vi "Configure Channel.vi"(0 "VISA resource name":refnum<visa-resource-name>, 1 "Enable Channel (T: Enable)":bool=TRUE, 2 "Input Impedance (0: 1M ohm)":u16(ring) items=["1M", "50"], 3 "Bandwidth (0: FULL)":u16(ring) items=["FULL", "500 MHz", "250 MHz", "150 MHz", "20 MHz"], 5 "Channel (0: Channel 1)":u16(ring) format="%#_5f" items=["Channel 1", "Channel 2", "Channel 3", "Channel 4", "Math 1", "Math 2", "Math 3", "Math 4", "Reference 1", "Reference 2", "Reference 3", "Reference 4"], 7 "Vertical Coupling (1: DC)":u16(ring)=1 items=["AC", "DC", "Ground"], 9 "Probe Attenuation (1.0)":dbl=1.0, 11 "error in (no error)":errorcluster, 12 "Vertical Range (10.0 V)":dbl=10.0, 13 "Vertical Offset (0.0 V)":dbl) -> (4 "VISA resource name out":refnum<visa-resource-name>, 15 "error out":errorcluster)   [LabVIEW 2015, in "Tektronix 7000 Series.lvlib"]
doc: "Configures the vertical properties of an oscilloscope for a specified channel. \n\n<B>Note:</B> \nThis VI does not configure channel settings for disabled channels."
uses:
  Tektronix 7000 Series.lvlib
panel:
  # "Input Channel Parameters"
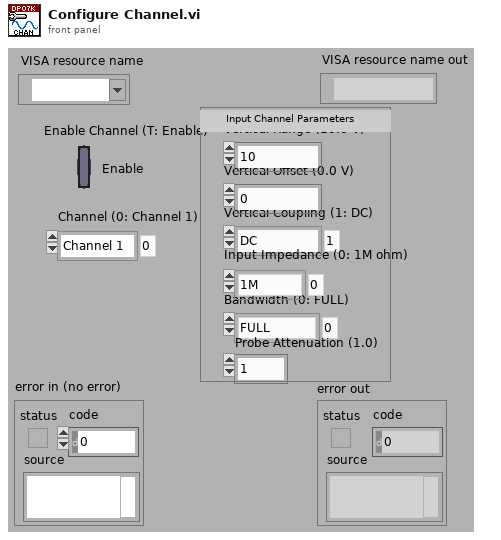
[diagram p1: front panel]
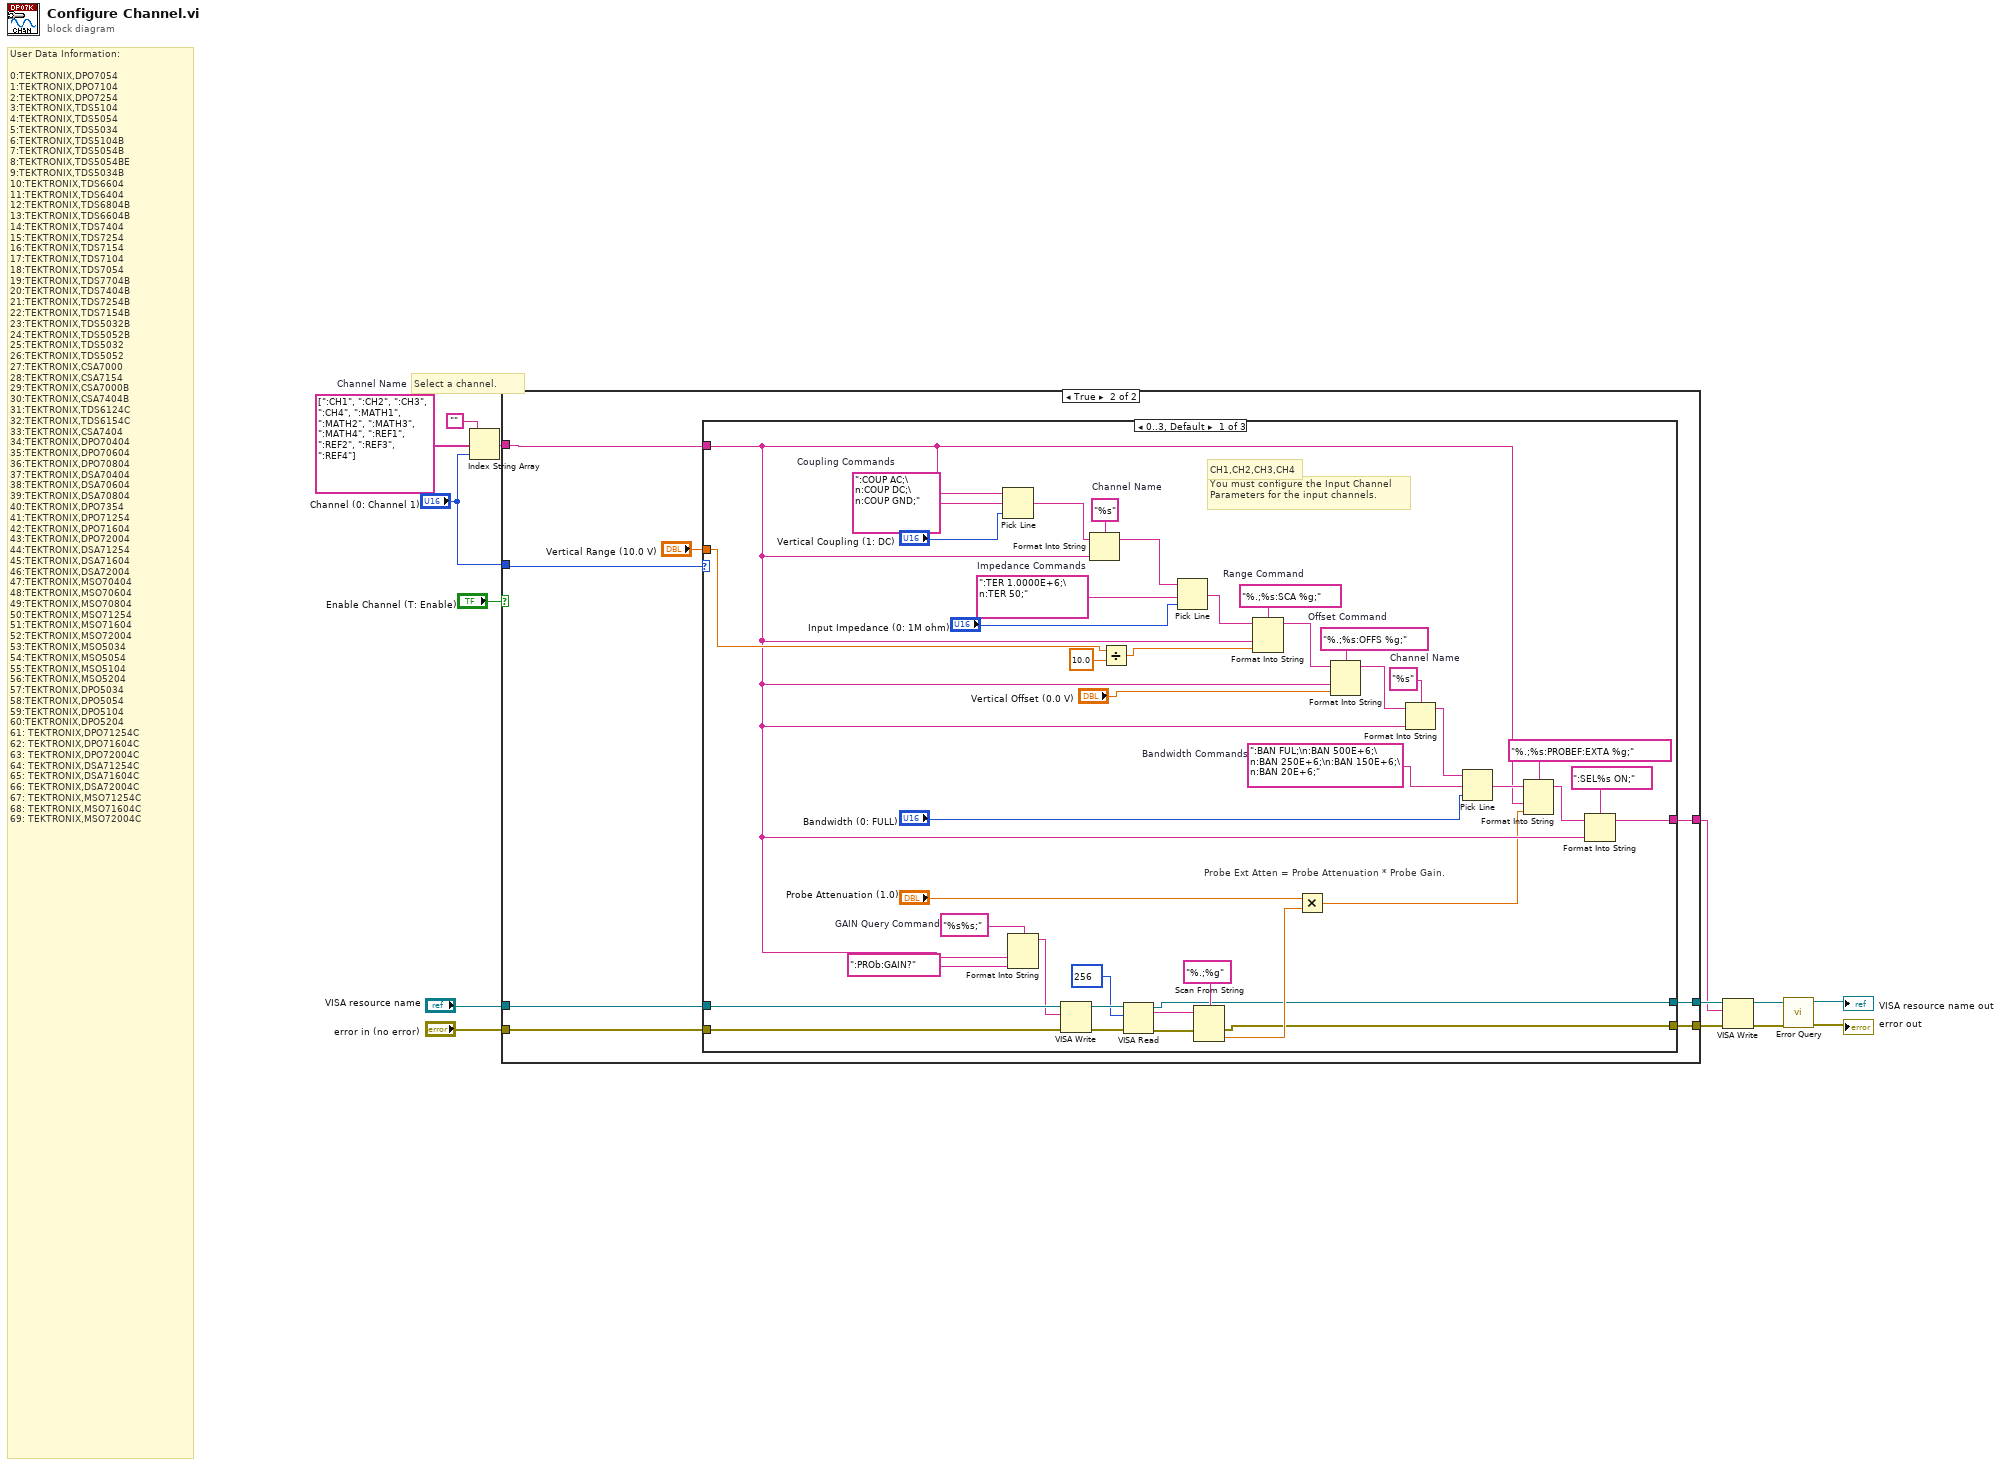
[diagram p0: block diagram]
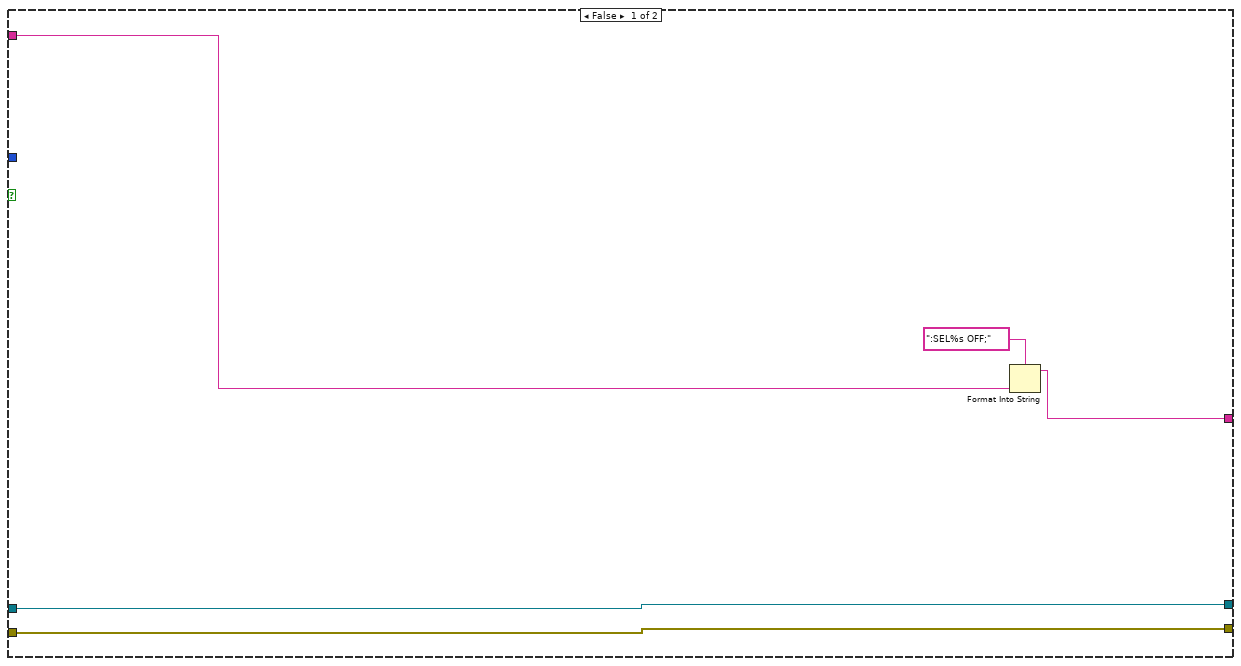
[diagram p2: hidden frame]
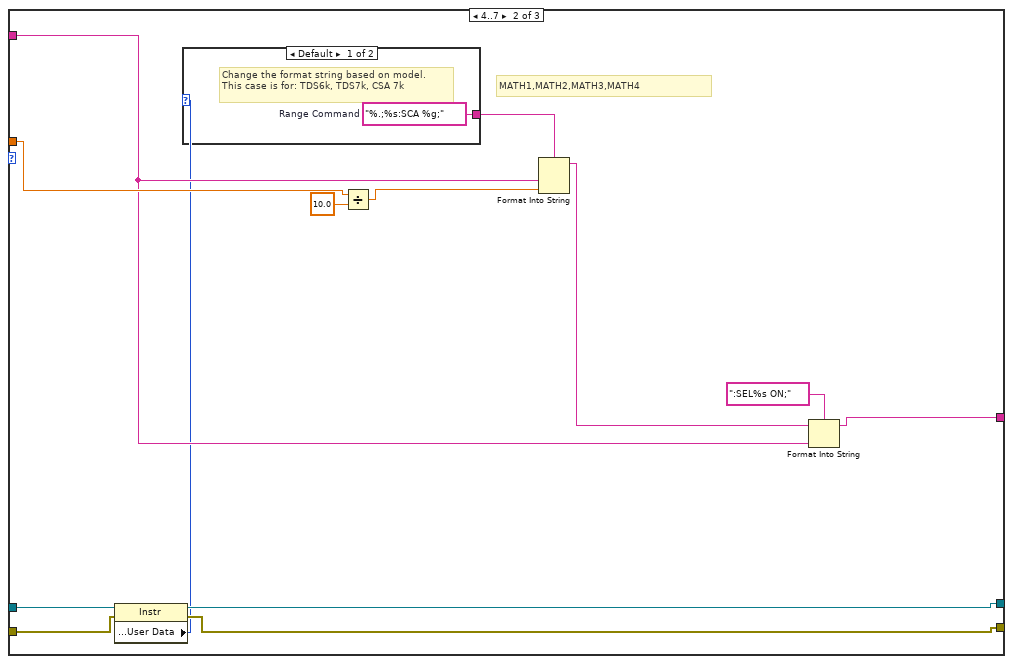
[diagram p3: hidden frame]
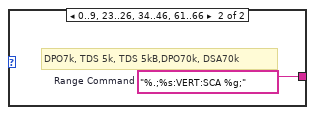
[diagram p4: hidden frame]
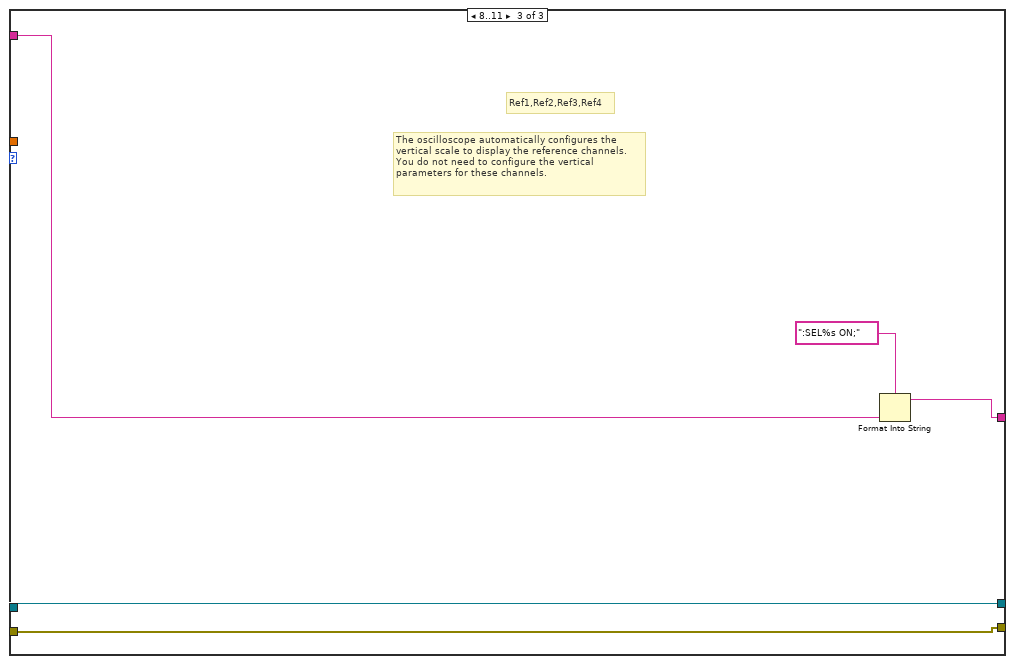
[diagram p5: hidden frame]
diagram:
  w11 = string[] [":CH1", ":CH2", ":CH3", ":CH4", ":MATH1", ":MATH2", ":MATH3", ":MATH4", ":REF1", ":REF2", ":REF3", ":REF4"]  # Channel Name
  # "User Data Information:\n\n0:TEKTRONIX,DPO7054\n1:TEKTRONIX,DPO7104\n2:TEKTRONIX,DPO7254\n3:TEKTRONIX,TDS5104\n4:TEKTRONIX,TDS5054\n5:TEKTRONIX,TDS5034\n6:TEKTRONIX,TDS5104B\n7:TEKTRONIX,TDS5054B\n8:TEKTRONIX,TDS5054BE\n9:TEKTRONIX,TDS5034B\n10:TEKTRONIX,TDS6604\n11:TEKTRONIX,TDS6404\n12:TEKTRONIX,TDS6804B\n13:TEKTRONIX,TDS6604B\n14:TEKTRONIX,TDS7404\n15:TEKTRONIX,TDS7254\n16:TEKTRONIX,TDS7154\n17:TEKTRONIX,TDS7104\n18:TEKTRONIX,TDS7054\n19:TEKTRONIX,TDS7704B\n20:TEKTRONIX,TDS7404B\n21:TEKTRONIX,TDS7254B\n22:TEKTRONIX,TDS7154B\n23:TEKTRONIX,TDS5032B\n24:TEKTRONIX,TDS5052B\n25:TEKTRONIX,TDS5032\n26:TEKTRONIX,TDS5052\n27:TEKTRONIX,CSA7000\n28:TEKTRONIX,CSA7154\n29:TEKTRONIX,CSA7000B\n30:TEKTRONIX,CSA7404B\n31:TEKTRONIX,TDS6124C\n32:TEKTRONIX,TDS6154C\n33:TEKTRONIX,CSA7404\n34:TEKTRONIX,DPO70404\n35:TEKTRONIX,DPO70604\n36:TEKTRONIX,DPO70804\n37:TEKTRONIX,DSA70404\n38:TEKTRONIX,DSA70604\n39:TEKTRONIX,DSA70804\n40:TEKTRONIX,DPO7354\n41:TEKTRONIX,DPO71254\n42:TEKTRONIX,DPO71604\n43:TEKTRONIX,DPO72004\n44:TEKTRONIX,DSA71254\n45:TEKTRONIX,DSA71604\n46:TEKTRONIX,DSA72004\n47:TEKTRONIX,MSO70404\n48:TEKTRONIX,MSO70604\n49:TEKTRONIX,MSO70804\n50:TEKTRONIX,MSO71254\n51:TEKTRONIX,MSO71604\n52:TEKTRONIX,MSO72004\n53:TEKTRONIX,MSO5034\n54:TEKTRONIX,MSO5054\n55:TEKTRONIX,MSO5104\n56:TEKTRONIX,MSO5204\n57:TEKTRONIX,DPO5034\n58:TEKTRONIX,DPO5054\n59:TEKTRONIX,DPO5104\n60:TEKTRONIX,DPO5204\n61: TEKTRONIX,DPO71254C\n62: TEKTRONIX,DPO71604C\n63: TEKTRONIX,DPO72004C\n64: TEKTRONIX,DSA71254C\n65: TEKTRONIX,DSA71604C\n66: TEKTRONIX,DSA72004C\n67: TEKTRONIX,MSO71254C\n68: TEKTRONIX,MSO71604C\n69: TEKTRONIX,MSO72004C"
  # "Select a channel."
  n1 = Index String Array(1:"Channel (0: Channel 1)", 2:w11, 3:"" ("Empty String Constant")) -> (0:w12:string)
  n2 = case shown="True" "Enable Channel (T: Enable)" {
    tunnel: w12 -> [w19 w27]
    tunnel: "Channel (0: Channel 1)" -> [_ w26]
    tunnel: "VISA resource name" -> [w16 w24]
    tunnel: "error in (no error)" -> [w15 w23]
    tunnel: [w16 w22] -> w3
    tunnel: [w15 w21] -> w2
    tunnel: [w17 w20] -> w1
    frame False {
      n3 = Format Into String(format string=":SEL%s OFF;", w19) -> (resulting string=w17:string)  [unwired: 2 in, 1 out]
    }
    frame True {
      n4 = case shown="0..3, Default" w26 {
        tunnel: w27 -> [w42 w77 w88]
        tunnel: "Vertical Range (10.0 V)" -> [w57 w80 _]
        tunnel: w24 -> [w45 w74 w86]
        tunnel: w23 -> [w44 w73 w85]
        tunnel: [w30 w72 w86] -> w22
        tunnel: [w29 w71 w85] -> w21
        tunnel: [w28 w76 w87] -> w20
        frame 0..3, Default {
          w41 = "%s%s;"  # GAIN Query Command
          w48 = "%.;%s:OFFS %g;"  # Offset Command
          w53 = "%s"  # Channel Name
          w54 = ":TER 1.0000E+6;\n:TER 50;"  # Impedance Commands
          w56 = "%.;%s:SCA %g;"  # Range Command
          w65 = ":BAN FUL;\n:BAN 500E+6;\n:BAN 250E+6;\n:BAN 150E+6;\n:BAN 20E+6;"  # Bandwidth Commands
          w67 = "%s"  # Channel Name
          w69 = ":COUP AC;\n:COUP DC;\n:COUP GND;"  # Coupling Commands
          # "CH1,CH2,CH3,CH4"
          # "Probe Ext Atten = Probe Attenuation * Probe Gain."
          # "You must configure the Input Channel\nParameters for the input channels."
          n5 = Pick Line(string ("")=w42, multi-line string=w69, line index="Vertical Coupling (1: DC)") -> (output string=w51:string)
          n6 = Format Into String(format string=w41, w42, ":PROb:GAIN?" ("write buffer")) -> (resulting string=w40:string)  [unwired: 2 in, 1 out]
          n7 = VISA Write(VISA resource name=w45, write buffer=w40, error in (no error)=w44) -> (VISA resource name out=w39:refnum<visa-resource-name>, error out=w38:errorcluster)  [unwired: 1 out]
          n8 = Format Into String(format string=w53, initial string=w51, w42) -> (resulting string=w52:string)  [unwired: 1 in, 1 out]
          n9 = Divide(x=w57, y=10.0) -> (x/y=w61:dbl)
          n10 = VISA Read(VISA resource name=w39, byte count=u32 256, error in (no error)=w38) -> (VISA resource name out=w30:refnum<visa-resource-name>, read buffer=w35:string, error out=w36:errorcluster)  [unwired: 1 out]
          n11 = Pick Line(string ("")=w52, multi-line string=w54, line index="Input Impedance (0: 1M ohm)") -> (output string=w50:string)
          n12 = Scan From String(format string="%.;%g", input string=w35, error in=w36) -> (error out=w29:errorcluster, output 1=w32:dbl)  [unwired: 2 in, 2 out]
          n13 = Format Into String(format string=w56, initial string=w50, w42, w61) -> (resulting string=w47:string)  [unwired: 1 in, 1 out]
          n14 = Multiply(x="Probe Attenuation (1.0)", y=w32) -> (x*y=w31:dbl)
          n15 = Format Into String(format string=w48, initial string=w47, w42, "Vertical Offset (0.0 V)") -> (resulting string=w46:string)  [unwired: 1 in, 1 out]
          n16 = Format Into String(format string=w67, initial string=w46, w42) -> (resulting string=w66:string)  [unwired: 1 in, 1 out]
          n17 = Pick Line(string ("")=w66, multi-line string=w65, line index="Bandwidth (0: FULL)") -> (output string=w59:string)
          n18 = Format Into String(format string="%.;%s:PROBEF:EXTA %g;", initial string=w59, w42, w31) -> (resulting string=w58:string)  [unwired: 1 in, 1 out]
          n19 = Format Into String(format string=":SEL%s ON;", initial string=w58, w42) -> (resulting string=w28:string)  [unwired: 1 in, 1 out]
        }
        frame 4..7 {
          # "MATH1,MATH2,MATH3,MATH4"
          n20 = property class="Instr"(reference=w74, error in=w73) -> (reference out=w72:refnum<visa-resource-name>, error out=w71:errorcluster, "General Settings:User Data"=w70:u32)
          n21 = case shown="Default" w70 {
            tunnel: [w83 w84] -> w75
            frame Default {
              w83 = "%.;%s:SCA %g;"  # Range Command
              # "Change the format string based on model.  This case is for: TDS6k, TDS7k, CSA 7k"
            }
            frame 0..9, 23..26, 34..46, 61..66 {
              w84 = "%.;%s:VERT:SCA %g;"  # Range Command
              # "DPO7k, TDS 5k, TDS 5kB,DPO70k, DSA70k"
            }
          }
          n22 = Divide(x=w80, y=10.0) -> (x/y=w79:dbl)
          n23 = Format Into String(format string=w75, w77, w79) -> (resulting string=w78:string)  [unwired: 2 in, 1 out]
          n24 = Format Into String(format string=":SEL%s ON;", initial string=w78, w77) -> (resulting string=w76:string)  [unwired: 1 in, 1 out]
        }
        frame 8..11 {
          # "Ref1,Ref2,Ref3,Ref4"
          # "The oscilloscope automatically configures the vertical scale to display the reference channels. You do not need to configure the vertical parameters for these channels."
          n25 = Format Into String(format string=":SEL%s ON;", w88) -> (resulting string=w87:string)  [unwired: 2 in, 1 out]
        }
      }
    }
  }
  n26 = VISA Write(VISA resource name=w3, write buffer=w1, error in (no error)=w2) -> (VISA resource name out=w7:refnum<visa-resource-name>, error out=w6:errorcluster)  [unwired: 1 out]
  n27 = call "Error Query.vi"("error in (no error)"=w6, "VISA resource name"=w7) -> ("error out"=→"error out":errorcluster, "VISA resource name out"=→"VISA resource name out":refnum<visa-resource-name>)  [unwired: 6 in, 2 out]
